vi "FilterTest.vi"() -> ()   [LabVIEW 2020]
uses:
  <vilib>/Analysis/NI_AALBase.lvlib
panel:
  out "Waveform Graph":dbl[](graph)
  in  "rank":i32=2
  out "Averaged Signal 2":dbl[][](graph)
  in  "IIR filter specifications":T1={"Topology"=enum."Inverse Chebyshev", "Type"=enum."Lowpass", "Order"=1, "Lower Fc"=200.0, "Upper Fc"=200.0, "PB Ripple"=1.0, "SB Attenuation"=60.0} {"PB Ripple" format="%0.2f"; "Lower Fc" format="%0.2p"; "SB Attenuation" format="%0.2f"; "Upper Fc" format="%0.2p"}
  in  "Averaged Signal":dbl[](graph)=[31043.4, 34409.6, 30819.0, 34477.0, 30985.2, 34271.2, 30989.0, 34591.2, 31072.0, 34203.0, 30965.4, 34623.6, 31139.8, 34474.6, 31205.0, 34699.8, 31342.2, 34472.2, 31520.6, 34814.8, 31607.6, 34590.8, 31554.4, 35030.6, 31724.4, 34790.4, 31766.4, 35113.2, 31833.2, 34895.0, 31781.8, 35128.6, 32061.2, 34963.4, 32087.4, 35312.8, 32192.8, 35005.6, 32195.8, 35307.6, 32121.2, 35115.6, 32372.0, 35402.4, 32447.2, 35111.0, 32363.6, 35401.8, 32516.6, 35177.8, 32461.2, 35455.2, 32690.6, 35223.4, 32550.0, 35483.6, 32659.0, 35172.0, 32680.4, 35440.2, 32641.2, 34996.0, 32580.8, 35466.8, 32532.6, 35018.2, 32612.0, 35220.6, 32536.6, 34893.8, 32595.6, 35166.0, 32728.4, 34913.6, 32565.6, 35167.8, 32675.4, 34964.8, 32723.2, 35165.0, 32695.4, 34960.6, 32695.8, 35227.2, 32674.6, 35060.2, 32798.8, 35394.8, 32790.8, 35081.6, 32832.8, 35327.2, 32948.6, 35045.2, 32864.8, 35380.2, 33012.6, 35145.6, 33055.8, 35391.4, 32960.0, 35209.2, 33042.8, 35468.2, 33160.0, 35163.4, 33140.4, 35500.8, 33105.4, 35285.8, 33202.2, 35491.0, 33254.0, 35290.8, 33298.4, 35563.0, 33372.2, 35287.8, 33251.0, 35437.0, 33336.8, 35425.2, 33365.2, 35612.8, 33584.2, 35460.6, 33380.8, 35730.4, 33462.0, 35456.4, 33493.2, 35601.8, 33610.4, 35584.0, 33581.0, 35758.0, 33583.0, 35626.8, 33702.4, 35875.2, 33654.2, 35600.4, 33760.4, 35783.0, 33666.0, 35623.0, 33705.6, 35855.6, 33698.2, 35623.4, 33656.8, 35916.2, 33801.8, 35643.4, 33728.4, 35912.2, 33744.2, 35796.2, 33804.8, 35986.6, 33828.6, 35786.4, 33816.4, 36038.0, 33980.2, 35871.8, 34036.8, 36118.0, 34016.6, 35839.4, 34044.8, 36143.8, 34088.4, 35881.2, 34111.0, 36165.8, 34032.0, 35972.8, 34241.4, 36200.0, 34099.0, 35995.6, 34219.2, 36219.2, 34154.4, 35979.0, 34120.8, 36109.8, 34110.6, 35882.6, 34153.2, 36244.6, 34186.2, 35980.8, 34236.6, 36332.0, 34163.8, 36053.0, 34239.8, 36204.2, 34189.0, 35884.4, 34147.2, 36074.8, 34064.4, 35786.4, 33955.6, 35946.4, 33855.2, 35641.4, 33814.8, 35919.8, 33813.2, 35571.8, 33747.6, 35710.4, 33812.2, 35396.2, 33701.4, 35667.6, 33684.8, 35273.8, 33663.0, 35490.4, 33441.6, 35146.0, 33612.6, 35427.0, 33401.4, 35062.0, 33401.0, 35418.2, 33486.2, 34992.6, 33350.6, 35287.8, 33412.6, 34974.6, 33332.2, 35310.4, 33478.0, 35004.8, 33494.0, 35403.4, 33572.8, 35131.2, 33434.0, 35453.8, 33638.8, 35305.4, 33671.4, 35570.2, 33676.8, 35383.2, 33706.8, 35710.8, 33885.2, 35545.0, 33937.4, 35727.0, 33878.2, 35471.6, 33769.4, 35665.4, 33948.0, 35422.6, 33820.2, 35618.4, 33932.6, 35452.2, 33871.0, 35649.2, 33854.0, 35396.8, 33770.4, 35653.0, 33830.8, 35393.8, 33729.6, 35664.4, 33896.2, 35239.2, 33758.4, 35671.4, 33829.0, 35487.2, 33782.4, 35591.4, 33723.4, 35304.8, 33751.4, 35521.6, 33595.8, 35215.0, 33548.0, 35446.4, 33600.4, 35174.0, 33632.4, 35493.8, 33532.2, 35136.0, 33540.6, 35512.2, 33478.0, 35171.0, 33438.4, 35365.6, 33595.6, 35116.4, 33521.0, 35328.8, 33673.8, 35129.4, 33599.0, 35323.4, 33497.6, 34948.6, 33487.8, 35219.0, 33424.6, 34975.0, 33451.0, 35217.0, 33395.0, 34885.2, 33403.8, 35105.8, 33364.0, 34837.0, 33278.0, 35101.6, 33384.6, 34837.8, 33283.2, 35072.8, 33374.6, 34772.4, 33330.0, 35120.2, 33308.6, 34832.6, 33305.4, 35071.8, 33221.6, 34916.4, 33288.2, 34979.0, 33156.6, 34680.0, 33149.8, 34953.2, 33129.4, 34585.2, 33234.0, 34890.4, 33107.8, 34643.4, 33135.6, 34887.2, 33082.6, 34578.6, 33178.0, 34821.4, 33134.8, 34512.2, 33099.8, 34850.6, 33047.4, 34519.6, 33048.8, 34798.8, 32964.6, 34450.8, 32972.4, 34710.2, 32946.4, 34437.4, 32892.4, 34630.6, 33026.6, 34314.6, 32949.6, 34517.0, 32944.6, 34174.6, 32984.6, 34603.6, 32897.8, 34301.4, 32929.0, 34636.4, 33032.4, 34427.2, 32871.8, 34739.8, 32982.8, 34262.0, 32905.0, 34596.0, 32919.2, 34273.2, 32901.8, 34517.6, 32854.6, 34225.4, 32862.0, 34597.0, 32924.2, 34212.4, 32938.0, 34547.0, 32778.4, 34266.4, 32787.6, 34538.4, 32854.4, 34250.0, 32881.6, 34533.4, 32813.2, 34113.0, 32761.2, 34452.6, 32736.4, 34124.0, 32756.6, 34418.2, 32817.0, 34180.8, 32853.8, 34465.4, 32685.6, 34142.6, 32851.8, 34304.8, 32750.2, 34070.2, 32788.6, 34445.0, 32766.4, 34060.2, 32766.2, 34366.8, 32825.0, 34092.2, 32709.4, 34372.2, 32723.4, 34120.8, 32710.2, 34260.0, 32774.8, 34018.2, 32687.8, 34209.8, 32669.0, 33952.6, 32627.4, 34267.8, 32696.6, 33909.4, 32602.8, 34225.4, 32615.6, 33885.4, 32536.2, 34113.8, 32518.8, 33767.6, 32413.0, 33967.8, 32395.6, 33596.2, 32384.8, 33889.4, 32376.2, 33567.2, 32340.4, 33830.4, 32268.6, 33551.0, 32278.8, 33864.8, 32279.0, 33491.4, 32218.8, 33726.8, 32104.4, 33431.4, 32127.6, 32906.0, 33684.4, 32099.0, 33392.2, 32150.2, 33592.4, 32101.4, 32581.4, 31985.6, 33582.8, 32112.4, 33319.0, 32156.2, 33612.2, 32049.0, 33207.4, 32108.6, 33516.8, 31922.2, 33181.0, 31973.0, 33477.2, 31897.4, 33121.0, 31966.4, 33242.8, 31821.0, 33111.2, 31824.6, 33315.4, 31755.2, 33100.0, 31690.4, 33217.8, 31710.2, 32939.2, 31668.0, 33086.4, 31705.4, 32810.2, 31552.0, 33084.4, 31609.2, 32778.8, 31612.4, 33022.4, 31562.2, 32677.4, 31530.8, 32849.2, 31434.8, 32662.4, 31331.6, 32943.0, 31442.4, 32655.0, 31485.2, 32851.8, 31343.4, 32555.6, 31366.2, 32769.0, 31328.0, 32441.8, 31203.0, 32714.4, 31221.2, 32453.6, 31061.0, 32634.4, 31072.4, 32205.8, 30966.0, 32439.6, 30964.0, 32050.6, 30807.4, 32179.0, 30746.6, 31968.2, 30688.8, 32170.0, 30729.4, 32012.8, 30733.2, 32115.6, 30709.6, 31896.8, 30654.6, 32175.4, 30706.2, 31823.8, 30626.8, 32018.0, 30380.4, 31758.8, 30587.8, 31931.8, 30369.0, 31628.2, 30477.0, 31877.2, 30343.8, 31622.8, 30385.4, 31859.2, 30311.6, 31495.2, 30364.4, 31784.4, 30252.0, 31428.6, 30136.6, 31587.2, 30220.8, 31349.8, 30039.4, 31524.6, 29964.4, 31166.2, 29995.8, 31405.0, 29894.8, 30999.8, 29799.2, 31287.4, 29873.6, 30993.6, 29819.2, 31344.0, 29870.6, 30966.0, 29843.4, 31113.6, 29766.6, 30869.2, 29680.2, 31171.4, 29720.6, 30751.6, 29572.2, 30986.0, 29578.4, 30737.6, 29610.6, 30841.6, 29598.4, 30551.0, 29486.8, 30872.4, 29422.0, 30548.4, 29330.2, 30709.0, 29272.6, 30424.8, 29249.0, 30503.2, 29116.0, 30391.0, 29087.8, 30498.4, 29149.4, 30212.4, 29062.0, 30403.8, 28951.2, 30084.6, 28806.4, 30293.6, 28931.0, 30073.6, 28904.0, 30203.6, 28830.0, 29917.0, 28796.6, 30162.2, 28750.0, 29823.0, 28723.2, 30060.0, 28729.2, 29759.8, 28638.8, 29976.8, 28655.6, 29711.6, 28603.4, 30012.6, 28494.4, 29752.8, 28533.4, 29826.0, 28490.8, 29626.2, 28406.6, 29723.0, 28377.4, 29411.0, 28305.4, 29631.4, 28167.0, 29312.0, 28229.0, 29566.4, 28152.2, 29329.6, 28218.6, 29499.6, 28068.6, 29242.4, 28091.0, 29464.4, 28107.8, 29251.4, 28145.0, 29394.8, 28063.4, 29075.6, 28124.8, 29317.8, 27963.2, 28990.0, 27962.6, 29302.2, 28030.4, 29091.6, 27994.4, 29272.0, 27996.8, 29133.8, 27946.8, 29311.0, 27983.0, 28990.2, 27935.0, 29296.6, 27810.4, 28933.8, 27940.4, 29260.2, 27928.8, 28890.8, 27893.2, 29183.4, 27830.4, 28874.0, 27804.8, 29142.6, 27873.2, 28869.4, 27842.6, 29132.8, 27820.6, 28851.2, 27856.6, 29085.0, 27801.2, 28862.0, 27749.4, 29002.8, 27678.4, 28799.4, 27694.8, 28951.2, 27718.8, 28749.6, 27619.4, 29007.4, 27614.2, 28813.8, 27725.8, 29067.4, 27638.4, 28699.0, 27715.6, 29013.8, 27637.8, 28679.2, 27681.4, 28921.6, 27555.6, 28672.0, 27538.6, 28880.8, 27443.8, 28663.4, 27493.6, 28894.0, 27504.8, 28482.0, 27332.2, 28796.4, 27456.4, 28585.0, 27348.4, 28691.0, 27312.2, 28420.6, 27363.6, 28725.0, 27408.8, 28514.0, 27300.2, 28755.4, 27373.8, 28453.0, 27344.6, 28582.6, 27345.4, 28455.0, 27339.2, 28547.8, 27229.0, 28280.2, 27174.8, 28516.4, 27203.2, 28327.0, 27271.8, 28470.8, 27118.8, 28431.4, 27240.4, 28482.2, 27093.8, 28229.2, 27202.6, 28459.4, 27187.4, 28249.0, 27194.8, 28448.0, 27120.0, 28267.6, 27094.6, 28483.8, 27159.6, 28187.6, 27127.8, 28342.0, 27095.2, 28186.6, 27018.4, 28343.6, 27029.2, 28213.8, 27016.2, 28393.0, 26957.2, 28080.8, 27021.6, 28293.6, 27017.6, 28050.6, 27022.6, 28332.0, 26964.4, 27997.0, 26913.8, 28223.6, 26760.0, 27951.6, 26831.0, 28176.2, 26829.4, 27997.8, 26799.0, 28108.2, 26789.4, 27873.8, 26797.6, 28138.6, 26703.6, 27730.8, 26815.6, 28007.8, 26627.6, 27711.6, 26711.2, 28044.0, 26697.2, 27938.2, 26648.4, 27976.8, 26627.4, 27727.0, 26719.6, 27900.2, 26600.2, 27619.8, 26522.6, 27820.6, 26525.2, 27567.8, 26540.2, 27800.4, 26377.4, 27469.4, 26345.6, 27698.8, 26386.0, 27396.2, 26370.4, 27560.4, 26276.2, 27372.4, 26202.6, 27541.4, 26204.8, 27235.8, 26183.2, 27430.6, 26175.4, 27223.2, 26137.8, 27416.8, 26083.8, 27222.2, 26184.4, 27499.6, 26170.2, 27160.6, 26232.4, 27370.0, 26033.0, 27117.4, 26111.8, 27364.0, 26012.4, 27054.6, 26072.4, 27333.8, 26062.6, 27103.4, 26061.8, 27245.6, 25926.2, 26979.2, 26053.8, 27269.4, 25869.8, 27002.6, 25973.4, 27319.8, 25855.2, 27058.0, 25920.2, 27305.6, 25961.6, 26975.6, 25918.4, 27127.4, 25962.2, 26937.8, 25787.4, 27073.2, 25785.6, 26846.2, 25735.4, 27072.6, 25644.6, 26684.0, 25791.6, 27188.8, 25723.2, 26884.2, 25806.4, 27086.2, 25820.2, 26770.6, 25743.2, 27086.8, 25749.6, 26830.4, 25758.8, 26947.8, 25588.8, 26694.0, 25702.2, 26869.6, 25615.0, 26549.2, 25585.6, 26979.2, 25564.0, 26609.4, 25571.4, 26804.0, 25448.2, 26464.8, 25413.2, 26769.2, 25410.4, 26485.6, 25382.4, 26627.6, 25387.2, 26461.0, 25333.4, 26527.2, 25391.6, 26360.2, 25368.0, 26650.4, 25276.6, 26318.2, 25338.4, 26602.8, 25267.4, 26292.4, 25306.4, 26557.8, 25200.6, 26339.2, 25290.6, 26530.0, 25255.2, 26305.6, 25235.0, 26373.6, 25083.8, 26174.4, 25105.0, 26243.2, 24977.4, 26040.2, 24889.2, 26098.4, 24836.2, 25965.4, 24866.6]
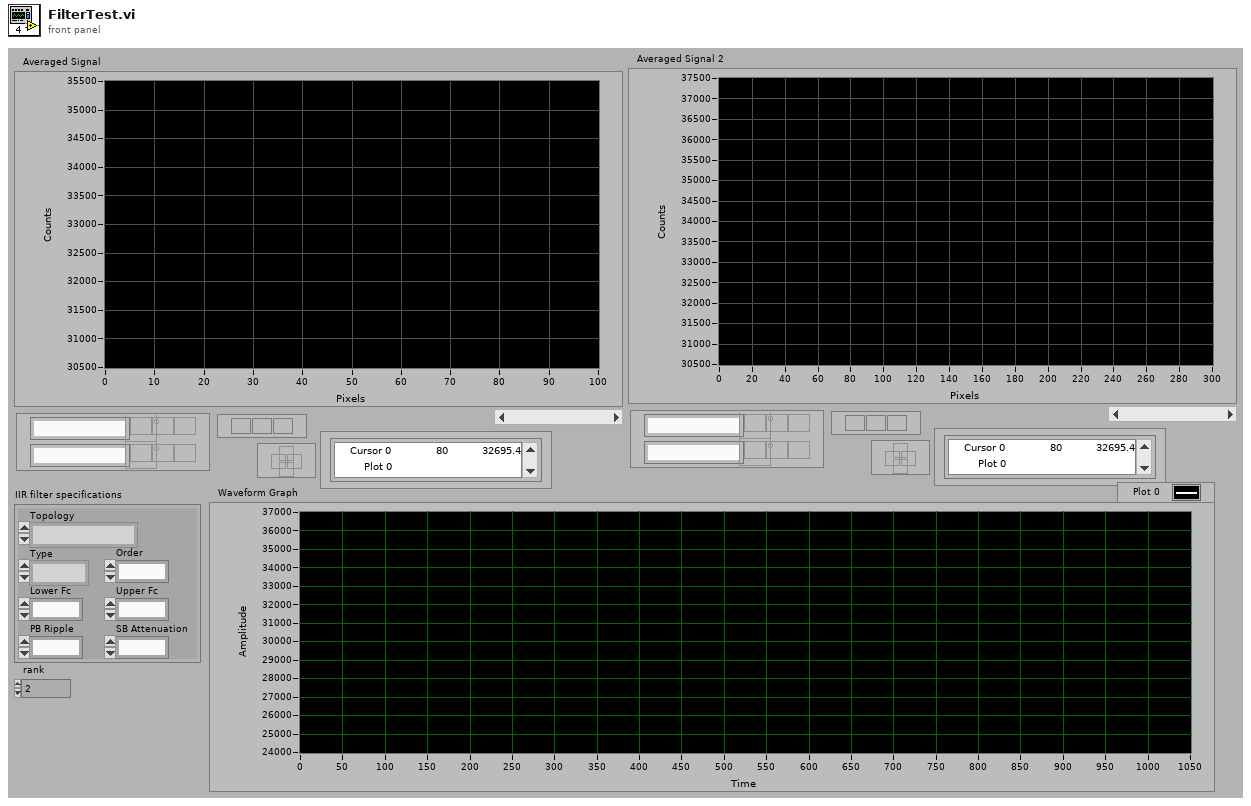
[diagram p1: front panel]
types:
  T1 = cluster{"Topology":enum16{"Off", "Butterworth", "Chebyshev", "Inverse Chebyshev", "Elliptic", "Bessel"}, "Type":enum16{"Lowpass", "Highpass", "Bandpass", "Bandstop"}, "Order":i32, "Lower Fc":dbl, "Upper Fc":dbl, "PB Ripple":dbl, "SB Attenuation":dbl}
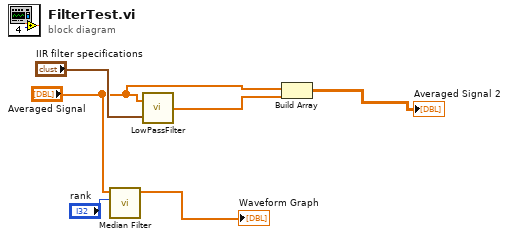
[diagram p0: block diagram]
diagram:
  n1 = call <vilib>:"Median Filter.vi"("left rank"="rank", "X"="Averaged Signal") -> ("Filtered X"=→"Waveform Graph":dbl[])  [unwired: 8 in, 1 out]
  n2 = call "LowPassFilter.vi"("IIR filter specifications"="IIR filter specifications", "Input Array"="Averaged Signal") -> ("output array"=w5:dbl[])
  n3 = Build Array("Averaged Signal", w5) -> (→"Averaged Signal 2":dbl[][])
